vi "加载配置.vi"(11 "默认配置选择":T1) -> (3 "配置表":T2={"设备类型"=enum."微站", "采配水模块类型"=enum."V4", "数据库类型"=enum."Access", "模块配置类型"=enum."单模块", "氨氮模块版本"=enum."V3", "总磷模块版本"=enum."V3", "总氮模块版本"=enum."V3", "CODMn模块版本"=enum."PLC版", "CODcr模块版本"=enum."斯坦道V3", "多参数模块版本"=enum."集成式多参", "加标回收模块版本"=enum."V4", "氨氮连接配置"={"启用"=TRUE, "连接类型"=enum."串口", "串口"="COM7", "IP"="192.168.1.202", "PORT"="502"}, "总磷连接配置"={"启用"=TRUE, "连接类型"=enum."串口", "串口"="COM5", "IP"="192.168.1.203", "PORT"="502"}, "总氮连接配置"={"启用"=TRUE, "连接类型"=enum."串口", "串口"="COM9", "IP"="192.168.1.204", "PORT"="502"}, "CODMn连接配置"={"启用"=TRUE, "连接类型"=enum."串口", "串口"="COM4", "IP"="192.168.1.201", "PORT"="502"}, "CODcr连接配置"={"启用"=FALSE, "连接类型"=enum."串口", "串口"="", "IP"="192.168.1.205", "PORT"="502"}, "多参数连接配置"={"启用"=TRUE, "连接类型"=enum."串口", "串口"="COM6", "IP"="192.168.1.206", "PORT"="502"}, "加标回收连接配置"={"启用"=TRUE, "连接类型"=enum."串口", "串口"="COM8", "IP"="192.168.1.207", "PORT"="502"}, "超标留样启用"=FALSE, "流量计启用"=FALSE, "河水净化启用"=FALSE, "进样类型"={"氨氮采样杯采样"=TRUE, "总磷采样杯采样"=TRUE, "总氮采样杯采样"=TRUE, "CODMn采样杯采样"=TRUE, "CODcr采样杯采样"=TRUE, "氟化物采样杯采样"=TRUE, "挥发酚采样杯采样"=FALSE}, "氟化物连接配置"={"启用"=FALSE, "连接类型"=enum."串口", "串口"="", "IP"="", "PORT"="502"}})   [LabVIEW 2016]
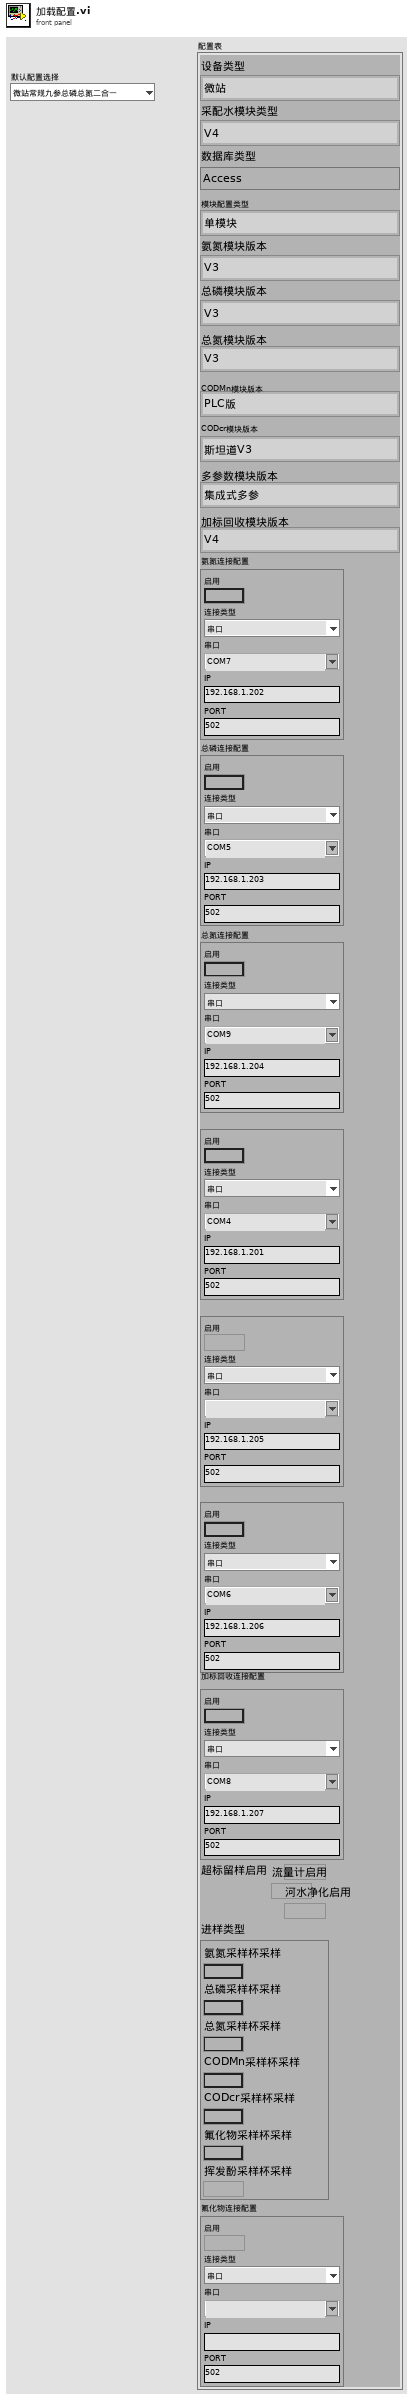
[diagram p1: front panel]
types:
  T1 = typedef "配置表选择.ctl" = enum16{"微站常规九参总磷总氮二合一", "微站常规八参氨氮总磷二合一", "微站常规九参", "微站常规八参", "固定站常规九参（TCP连接）", "固定站常规九参（串口连接）", "浮船常规九参总磷总氮二合一", "浮船常规九参"}
  T2 = typedef "模块配置表.ctl" = cluster{"设备类型":T3, "采配水模块类型":T4, "数据库类型":T5, "模块配置类型":T6, "氨氮模块版本":T7, "总磷模块版本":T7, "总氮模块版本":T7, "CODMn模块版本":T8, "CODcr模块版本":T9, "多参数模块版本":T10, "加标回收模块版本":T11, "氨氮连接配置":T12, "总磷连接配置":T12, "总氮连接配置":T12, "CODMn连接配置":T12, "CODcr连接配置":T12, "多参数连接配置":T12, "加标回收连接配置":T12, "超标留样启用":bool, "流量计启用":bool, "河水净化启用":bool, "进样类型":cluster{"氨氮采样杯采样":bool, "总磷采样杯采样":bool, "总氮采样杯采样":bool, "CODMn采样杯采样":bool, "CODcr采样杯采样":bool, "氟化物采样杯采样":bool, "挥发酚采样杯采样":bool}, "氟化物连接配置":T12}
  T3 = typedef "设备类型.ctl" = enum16{"微站", "固定站", "浮船"}
  T4 = typedef "采配水类型.ctl" = enum16{"V1", "V2", "V3", "V4", "室内V1", "室内V2", "固定站V1", "固定站V2", "浮船V1", "浮船V2"}
  T5 = typedef "数据库类型.ctl" = enum16{"Access", "SQLite"}
  T6 = typedef "模块配置类型.ctl" = enum16{"单模块", "总磷总氮二合一模块", "氨氮总磷二合一模块"}
  T7 = typedef "氨氮总磷总氮模块版本.ctl" = enum16{"V2", "V3"}
  T8 = typedef "CODMn模块版本.ctl" = enum16{"PLC版", "单片机版", "通用流路版本"}
  T9 = typedef "CODcr模块版本.ctl" = enum16{"斯坦道V3", "点创"}
  T10 = typedef "多参数模块版本.ctl" = enum16{"原位多参数", "集成式多参"}
  T11 = typedef "加标回收模块版本.ctl" = enum16{"V1", "V2", "V4"}
  T12 = typedef "连接配置.ctl" = cluster{"启用":bool, "连接类型":enum16{"串口", "TCP"}, "串口":string, "IP":string, "PORT":string}
  T13 = cluster{"微站常规九参总磷总氮二合一配置表":T2, "微站常规八参氨氮总磷二合一配置表":T2, "微站常规九参配置表":T2, "微站常规八参配置表":T2, "固定站常规九参配置表（TCP）":T2, "浮船常规九参总磷总氮二合一配置表":T2, "浮船常规九参配置表":T2, "固定站常规九参配置表（串口）":T2}
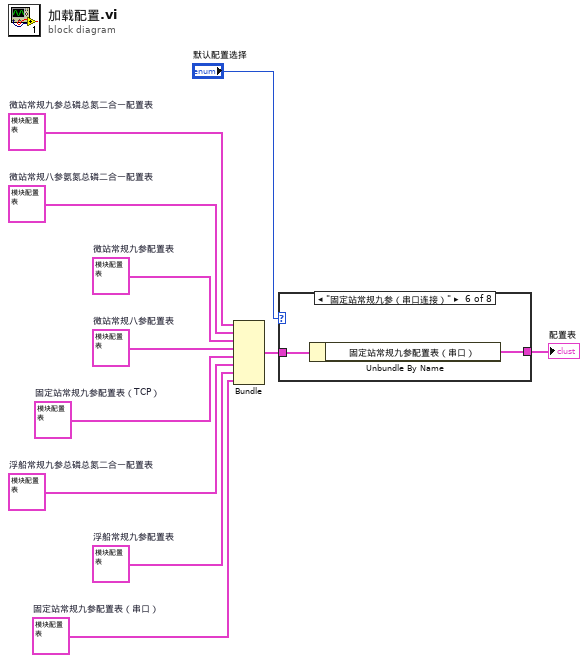
[diagram p0: block diagram]
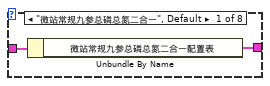
[diagram p2: hidden frame]
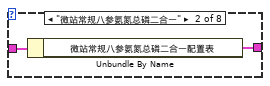
[diagram p3: hidden frame]
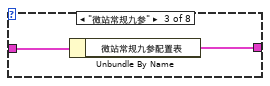
[diagram p4: hidden frame]
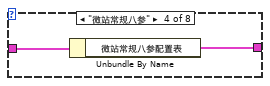
[diagram p5: hidden frame]
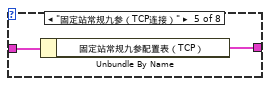
[diagram p6: hidden frame]
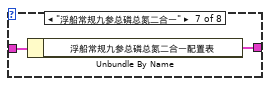
[diagram p7: hidden frame]
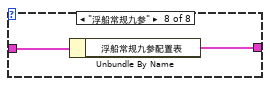
[diagram p8: hidden frame]
diagram:
  w1 = T2 {"设备类型"=enum."固定站", "采配水模块类型"=enum."固定站V2", "数据库类型"=enum."Access", "模块配置类型"=enum."单模块", "氨氮模块版本"=enum."V3", "总磷模块版本"=enum."V3", "总氮模块版本"=enum."V3", "CODMn模块版本"=enum."单片机版", "CODcr模块版本"=enum."斯坦道V3", "多参数模块版本"=enum."集成式多参", "加标回收模块版本"=enum."V4", "氨氮连接配置"={"启用"=TRUE, "连接类型"=enum."串口", "串口"="COM7", "IP"="192.168.1.202", "PORT"="502"}, "总磷连接配置"={"启用"=TRUE, "连接类型"=enum."串口", "串口"="COM5", "IP"="192.168.1.203", "PORT"="502"}, "总氮连接配置"={"启用"=TRUE, "连接类型"=enum."串口", "串口"="COM9", "IP"="192.168.1.204", "PORT"="502"}, "CODMn连接配置"={"启用"=TRUE, "连接类型"=enum."串口", "串口"="COM4", "IP"="192.168.1.201", "PORT"="502"}, "CODcr连接配置"={"启用"=FALSE, "连接类型"=enum."串口", "串口"="", "IP"="192.168.1.205", "PORT"="502"}, "多参数连接配置"={"启用"=TRUE, "连接类型"=enum."串口", "串口"="COM6", "IP"="192.168.1.206", "PORT"="502"}, "加标回收连接配置"={"启用"=TRUE, "连接类型"=enum."串口", "串口"="COM8", "IP"="192.168.1.207", "PORT"="502"}, "超标留样启用"=FALSE, "流量计启用"=FALSE, "河水净化启用"=FALSE, "进样类型"={"氨氮采样杯采样"=TRUE, "总磷采样杯采样"=TRUE, "总氮采样杯采样"=TRUE, "CODMn采样杯采样"=TRUE, "CODcr采样杯采样"=TRUE, "氟化物采样杯采样"=FALSE, "挥发酚采样杯采样"=FALSE}, "氟化物连接配置"={"启用"=FALSE, "连接类型"=enum."串口", "串口"="", "IP"="", "PORT"="502"}}  # 固定站常规九参配置表（串口）
  w8 = T2 {"设备类型"=enum."微站", "采配水模块类型"=enum."V4", "数据库类型"=enum."Access", "模块配置类型"=enum."单模块", "氨氮模块版本"=enum."V3", "总磷模块版本"=enum."V3", "总氮模块版本"=enum."V3", "CODMn模块版本"=enum."单片机版", "CODcr模块版本"=enum."斯坦道V3", "多参数模块版本"=enum."集成式多参", "加标回收模块版本"=enum."V4", "氨氮连接配置"={"启用"=TRUE, "连接类型"=enum."串口", "串口"="COM7", "IP"="192.168.1.202", "PORT"="502"}, "总磷连接配置"={"启用"=TRUE, "连接类型"=enum."串口", "串口"="COM5", "IP"="192.168.1.203", "PORT"="502"}, "总氮连接配置"={"启用"=FALSE, "连接类型"=enum."串口", "串口"="COM9", "IP"="192.168.1.204", "PORT"="502"}, "CODMn连接配置"={"启用"=TRUE, "连接类型"=enum."串口", "串口"="COM4", "IP"="192.168.1.201", "PORT"="502"}, "CODcr连接配置"={"启用"=FALSE, "连接类型"=enum."串口", "串口"="", "IP"="192.168.1.205", "PORT"="502"}, "多参数连接配置"={"启用"=TRUE, "连接类型"=enum."串口", "串口"="COM6", "IP"="192.168.1.206", "PORT"="502"}, "加标回收连接配置"={"启用"=TRUE, "连接类型"=enum."串口", "串口"="COM8", "IP"="192.168.1.207", "PORT"="502"}, "超标留样启用"=FALSE, "流量计启用"=FALSE, "河水净化启用"=FALSE, "进样类型"={"氨氮采样杯采样"=TRUE, "总磷采样杯采样"=TRUE, "总氮采样杯采样"=FALSE, "CODMn采样杯采样"=TRUE, "CODcr采样杯采样"=TRUE, "氟化物采样杯采样"=FALSE, "挥发酚采样杯采样"=FALSE}, "氟化物连接配置"={"启用"=FALSE, "连接类型"=enum."串口", "串口"="", "IP"="", "PORT"="502"}}  # 微站常规八参配置表
  w10 = T2 {"设备类型"=enum."微站", "采配水模块类型"=enum."V4", "数据库类型"=enum."Access", "模块配置类型"=enum."氨氮总磷二合一模块", "氨氮模块版本"=enum."V3", "总磷模块版本"=enum."V3", "总氮模块版本"=enum."V3", "CODMn模块版本"=enum."PLC版", "CODcr模块版本"=enum."斯坦道V3", "多参数模块版本"=enum."集成式多参", "加标回收模块版本"=enum."V4", "氨氮连接配置"={"启用"=TRUE, "连接类型"=enum."串口", "串口"="COM7", "IP"="192.168.1.202", "PORT"="502"}, "总磷连接配置"={"启用"=FALSE, "连接类型"=enum."串口", "串口"="COM5", "IP"="192.168.1.203", "PORT"="502"}, "总氮连接配置"={"启用"=FALSE, "连接类型"=enum."串口", "串口"="COM9", "IP"="192.168.1.204", "PORT"="502"}, "CODMn连接配置"={"启用"=TRUE, "连接类型"=enum."串口", "串口"="COM4", "IP"="192.168.1.201", "PORT"="502"}, "CODcr连接配置"={"启用"=FALSE, "连接类型"=enum."串口", "串口"="", "IP"="192.168.1.205", "PORT"="502"}, "多参数连接配置"={"启用"=TRUE, "连接类型"=enum."串口", "串口"="COM6", "IP"="192.168.1.206", "PORT"="502"}, "加标回收连接配置"={"启用"=TRUE, "连接类型"=enum."串口", "串口"="COM8", "IP"="192.168.1.207", "PORT"="502"}, "超标留样启用"=FALSE, "流量计启用"=FALSE, "河水净化启用"=FALSE, "进样类型"={"氨氮采样杯采样"=TRUE, "总磷采样杯采样"=TRUE, "总氮采样杯采样"=FALSE, "CODMn采样杯采样"=FALSE, "CODcr采样杯采样"=FALSE, "氟化物采样杯采样"=FALSE, "挥发酚采样杯采样"=FALSE}, "氟化物连接配置"={"启用"=FALSE, "连接类型"=enum."串口", "串口"="", "IP"="", "PORT"="502"}}  # 微站常规八参氨氮总磷二合一配置表
  w11 = T2 {"设备类型"=enum."微站", "采配水模块类型"=enum."V4", "数据库类型"=enum."Access", "模块配置类型"=enum."总磷总氮二合一模块", "氨氮模块版本"=enum."V3", "总磷模块版本"=enum."V3", "总氮模块版本"=enum."V3", "CODMn模块版本"=enum."PLC版", "CODcr模块版本"=enum."斯坦道V3", "多参数模块版本"=enum."集成式多参", "加标回收模块版本"=enum."V4", "氨氮连接配置"={"启用"=TRUE, "连接类型"=enum."串口", "串口"="COM7", "IP"="192.168.1.202", "PORT"="502"}, "总磷连接配置"={"启用"=TRUE, "连接类型"=enum."串口", "串口"="COM5", "IP"="192.168.1.203", "PORT"="502"}, "总氮连接配置"={"启用"=FALSE, "连接类型"=enum."串口", "串口"="COM9", "IP"="192.168.1.204", "PORT"="502"}, "CODMn连接配置"={"启用"=TRUE, "连接类型"=enum."串口", "串口"="COM4", "IP"="192.168.1.201", "PORT"="502"}, "CODcr连接配置"={"启用"=FALSE, "连接类型"=enum."串口", "串口"="", "IP"="192.168.1.205", "PORT"="502"}, "多参数连接配置"={"启用"=TRUE, "连接类型"=enum."串口", "串口"="COM6", "IP"="192.168.1.206", "PORT"="502"}, "加标回收连接配置"={"启用"=TRUE, "连接类型"=enum."串口", "串口"="COM8", "IP"="192.168.1.207", "PORT"="502"}, "超标留样启用"=FALSE, "流量计启用"=FALSE, "河水净化启用"=FALSE, "进样类型"={"氨氮采样杯采样"=TRUE, "总磷采样杯采样"=TRUE, "总氮采样杯采样"=TRUE, "CODMn采样杯采样"=TRUE, "CODcr采样杯采样"=TRUE, "氟化物采样杯采样"=TRUE, "挥发酚采样杯采样"=FALSE}, "氟化物连接配置"={"启用"=FALSE, "连接类型"=enum."串口", "串口"="", "IP"="", "PORT"="502"}}  # 微站常规九参总磷总氮二合一配置表
  w6 = T2 {"设备类型"=enum."浮船", "采配水模块类型"=enum."浮船V2", "数据库类型"=enum."Access", "模块配置类型"=enum."总磷总氮二合一模块", "氨氮模块版本"=enum."V3", "总磷模块版本"=enum."V3", "总氮模块版本"=enum."V3", "CODMn模块版本"=enum."PLC版", "CODcr模块版本"=enum."斯坦道V3", "多参数模块版本"=enum."集成式多参", "加标回收模块版本"=enum."V4", "氨氮连接配置"={"启用"=TRUE, "连接类型"=enum."串口", "串口"="COM7", "IP"="192.168.1.202", "PORT"="502"}, "总磷连接配置"={"启用"=TRUE, "连接类型"=enum."串口", "串口"="COM5", "IP"="192.168.1.203", "PORT"="502"}, "总氮连接配置"={"启用"=FALSE, "连接类型"=enum."串口", "串口"="COM9", "IP"="192.168.1.204", "PORT"="502"}, "CODMn连接配置"={"启用"=TRUE, "连接类型"=enum."串口", "串口"="COM4", "IP"="192.168.1.201", "PORT"="502"}, "CODcr连接配置"={"启用"=FALSE, "连接类型"=enum."串口", "串口"="", "IP"="192.168.1.205", "PORT"="502"}, "多参数连接配置"={"启用"=TRUE, "连接类型"=enum."串口", "串口"="COM6", "IP"="192.168.1.206", "PORT"="502"}, "加标回收连接配置"={"启用"=FALSE, "连接类型"=enum."串口", "串口"="COM8", "IP"="192.168.1.207", "PORT"="502"}, "超标留样启用"=FALSE, "流量计启用"=FALSE, "河水净化启用"=FALSE, "进样类型"={"氨氮采样杯采样"=FALSE, "总磷采样杯采样"=FALSE, "总氮采样杯采样"=FALSE, "CODMn采样杯采样"=FALSE, "CODcr采样杯采样"=FALSE, "氟化物采样杯采样"=FALSE, "挥发酚采样杯采样"=FALSE}, "氟化物连接配置"={"启用"=FALSE, "连接类型"=enum."串口", "串口"="", "IP"="", "PORT"="502"}}  # 浮船常规九参总磷总氮二合一配置表
  w5 = T2 {"设备类型"=enum."浮船", "采配水模块类型"=enum."浮船V2", "数据库类型"=enum."Access", "模块配置类型"=enum."单模块", "氨氮模块版本"=enum."V3", "总磷模块版本"=enum."V3", "总氮模块版本"=enum."V3", "CODMn模块版本"=enum."PLC版", "CODcr模块版本"=enum."斯坦道V3", "多参数模块版本"=enum."集成式多参", "加标回收模块版本"=enum."V4", "氨氮连接配置"={"启用"=TRUE, "连接类型"=enum."串口", "串口"="COM7", "IP"="192.168.1.202", "PORT"="502"}, "总磷连接配置"={"启用"=TRUE, "连接类型"=enum."串口", "串口"="COM5", "IP"="192.168.1.203", "PORT"="502"}, "总氮连接配置"={"启用"=TRUE, "连接类型"=enum."串口", "串口"="COM9", "IP"="192.168.1.204", "PORT"="502"}, "CODMn连接配置"={"启用"=TRUE, "连接类型"=enum."串口", "串口"="COM4", "IP"="192.168.1.201", "PORT"="502"}, "CODcr连接配置"={"启用"=FALSE, "连接类型"=enum."串口", "串口"="", "IP"="192.168.1.205", "PORT"="502"}, "多参数连接配置"={"启用"=TRUE, "连接类型"=enum."串口", "串口"="COM6", "IP"="192.168.1.206", "PORT"="502"}, "加标回收连接配置"={"启用"=FALSE, "连接类型"=enum."串口", "串口"="COM8", "IP"="192.168.1.207", "PORT"="502"}, "超标留样启用"=FALSE, "流量计启用"=FALSE, "河水净化启用"=FALSE, "进样类型"={"氨氮采样杯采样"=FALSE, "总磷采样杯采样"=FALSE, "总氮采样杯采样"=FALSE, "CODMn采样杯采样"=FALSE, "CODcr采样杯采样"=FALSE, "氟化物采样杯采样"=FALSE, "挥发酚采样杯采样"=FALSE}, "氟化物连接配置"={"启用"=FALSE, "连接类型"=enum."串口", "串口"="", "IP"="", "PORT"="502"}}  # 浮船常规九参配置表
  w7 = T2 {"设备类型"=enum."固定站", "采配水模块类型"=enum."固定站V2", "数据库类型"=enum."Access", "模块配置类型"=enum."单模块", "氨氮模块版本"=enum."V3", "总磷模块版本"=enum."V3", "总氮模块版本"=enum."V3", "CODMn模块版本"=enum."单片机版", "CODcr模块版本"=enum."斯坦道V3", "多参数模块版本"=enum."集成式多参", "加标回收模块版本"=enum."V4", "氨氮连接配置"={"启用"=TRUE, "连接类型"=enum."TCP", "串口"="COM7", "IP"="192.168.1.202", "PORT"="502"}, "总磷连接配置"={"启用"=TRUE, "连接类型"=enum."TCP", "串口"="COM5", "IP"="192.168.1.203", "PORT"="502"}, "总氮连接配置"={"启用"=TRUE, "连接类型"=enum."TCP", "串口"="COM9", "IP"="192.168.1.204", "PORT"="502"}, "CODMn连接配置"={"启用"=TRUE, "连接类型"=enum."TCP", "串口"="COM4", "IP"="192.168.1.201", "PORT"="502"}, "CODcr连接配置"={"启用"=FALSE, "连接类型"=enum."TCP", "串口"="", "IP"="192.168.1.205", "PORT"="502"}, "多参数连接配置"={"启用"=TRUE, "连接类型"=enum."TCP", "串口"="COM6", "IP"="192.168.1.206", "PORT"="502"}, "加标回收连接配置"={"启用"=TRUE, "连接类型"=enum."TCP", "串口"="COM8", "IP"="192.168.1.207", "PORT"="502"}, "超标留样启用"=FALSE, "流量计启用"=FALSE, "河水净化启用"=FALSE, "进样类型"={"氨氮采样杯采样"=TRUE, "总磷采样杯采样"=TRUE, "总氮采样杯采样"=TRUE, "CODMn采样杯采样"=TRUE, "CODcr采样杯采样"=TRUE, "氟化物采样杯采样"=FALSE, "挥发酚采样杯采样"=FALSE}, "氟化物连接配置"={"启用"=FALSE, "连接类型"=enum."串口", "串口"="", "IP"="", "PORT"="502"}}  # 固定站常规九参配置表（TCP）
  w9 = T2 {"设备类型"=enum."微站", "采配水模块类型"=enum."V4", "数据库类型"=enum."Access", "模块配置类型"=enum."单模块", "氨氮模块版本"=enum."V3", "总磷模块版本"=enum."V3", "总氮模块版本"=enum."V3", "CODMn模块版本"=enum."单片机版", "CODcr模块版本"=enum."斯坦道V3", "多参数模块版本"=enum."集成式多参", "加标回收模块版本"=enum."V4", "氨氮连接配置"={"启用"=TRUE, "连接类型"=enum."串口", "串口"="COM7", "IP"="192.168.1.202", "PORT"="502"}, "总磷连接配置"={"启用"=TRUE, "连接类型"=enum."串口", "串口"="COM5", "IP"="192.168.1.203", "PORT"="502"}, "总氮连接配置"={"启用"=TRUE, "连接类型"=enum."串口", "串口"="COM9", "IP"="192.168.1.204", "PORT"="502"}, "CODMn连接配置"={"启用"=TRUE, "连接类型"=enum."串口", "串口"="COM4", "IP"="192.168.1.201", "PORT"="502"}, "CODcr连接配置"={"启用"=FALSE, "连接类型"=enum."串口", "串口"="", "IP"="192.168.1.205", "PORT"="502"}, "多参数连接配置"={"启用"=TRUE, "连接类型"=enum."串口", "串口"="COM6", "IP"="192.168.1.206", "PORT"="502"}, "加标回收连接配置"={"启用"=TRUE, "连接类型"=enum."串口", "串口"="COM8", "IP"="192.168.1.207", "PORT"="502"}, "超标留样启用"=FALSE, "流量计启用"=FALSE, "河水净化启用"=FALSE, "进样类型"={"氨氮采样杯采样"=TRUE, "总磷采样杯采样"=TRUE, "总氮采样杯采样"=TRUE, "CODMn采样杯采样"=TRUE, "CODcr采样杯采样"=TRUE, "氟化物采样杯采样"=TRUE, "挥发酚采样杯采样"=FALSE}, "氟化物连接配置"={"启用"=FALSE, "连接类型"=enum."串口", "串口"="", "IP"="", "PORT"="502"}}  # 微站常规九参配置表
  n1 = Bundle ("捆绑")("微站常规九参总磷总氮二合一配置表"=w11, "微站常规八参氨氮总磷二合一配置表"=w10, "微站常规九参配置表"=w9, "微站常规八参配置表"=w8, "固定站常规九参配置表（TCP）"=w7, "浮船常规九参总磷总氮二合一配置表"=w6, "浮船常规九参配置表"=w5, "固定站常规九参配置表（串口）"=w1) -> (w3:T13)  [unwired: 1 in]
  n2 = case shown="\"固定站常规九参（串口连接）\"" "默认配置选择" {
    tunnel: w3 -> [w13 w15 w17 w19 w21 w23 w25 w27]
    tunnel: [w12 w14 w16 w18 w20 w22 w24 w26] -> w2
    frame "微站常规九参总磷总氮二合一", Default {
      n3 = Unbundle By Name(w13) -> ("微站常规九参总磷总氮二合一配置表"=w12:T2)
    }
    frame "微站常规八参氨氮总磷二合一" {
      n4 = Unbundle By Name(w15) -> ("微站常规八参氨氮总磷二合一配置表"=w14:T2)
    }
    frame "微站常规九参" {
      n5 = Unbundle By Name(w17) -> ("微站常规九参配置表"=w16:T2)
    }
    frame "微站常规八参" {
      n6 = Unbundle By Name(w19) -> ("微站常规八参配置表"=w18:T2)
    }
    frame "固定站常规九参（TCP连接）" {
      n7 = Unbundle By Name(w21) -> ("固定站常规九参配置表（TCP）"=w20:T2)
    }
    frame "固定站常规九参（串口连接）" {
      n8 = Unbundle By Name(w23) -> ("固定站常规九参配置表（串口）"=w22:T2)
    }
    frame "浮船常规九参总磷总氮二合一" {
      n9 = Unbundle By Name(w25) -> ("浮船常规九参总磷总氮二合一配置表"=w24:T2)
    }
    frame "浮船常规九参" {
      n10 = Unbundle By Name(w27) -> ("浮船常规九参配置表"=w26:T2)
    }
  }
  "配置表" <- w2
